vi "ReadPoints.vi"(8 "error in (no error)":errorcluster caption="错误输入（无错误）", 10 "工站":string, 11 "机种":string) -> (0 "error out":errorcluster caption="错误输出", 1 "Calcu":dbl[](array[numeric]), 2 "points":dbl[][](array[numeric]), 3 "Robot":cluster{"X":dbl, "Y":dbl}, 4 "RefMove":cluster{"X":dbl, "Y":dbl}, 5 "参考位":string)   [LabVIEW 2016]
uses:
  <vilib>/Utility/config.llb/Read Key (String).vi
  <vilib>/Utility/config.llb/NI_LVConfig.lvlib
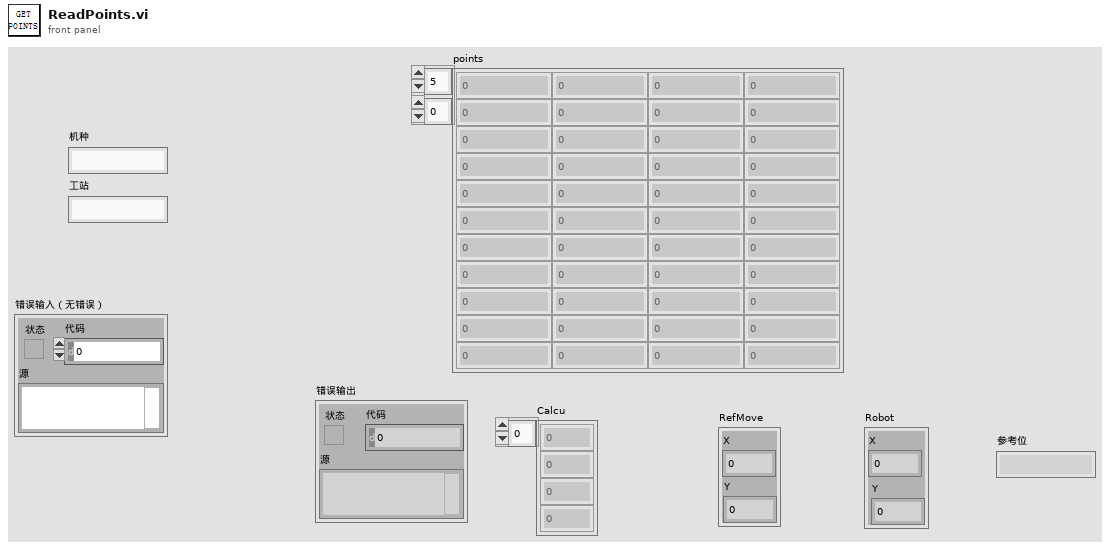
[diagram p1: front panel]
types:
  T1 = typedef "NI_LVConfig.lvlib/Config Data RefNum.ctl" = refnum<k1>
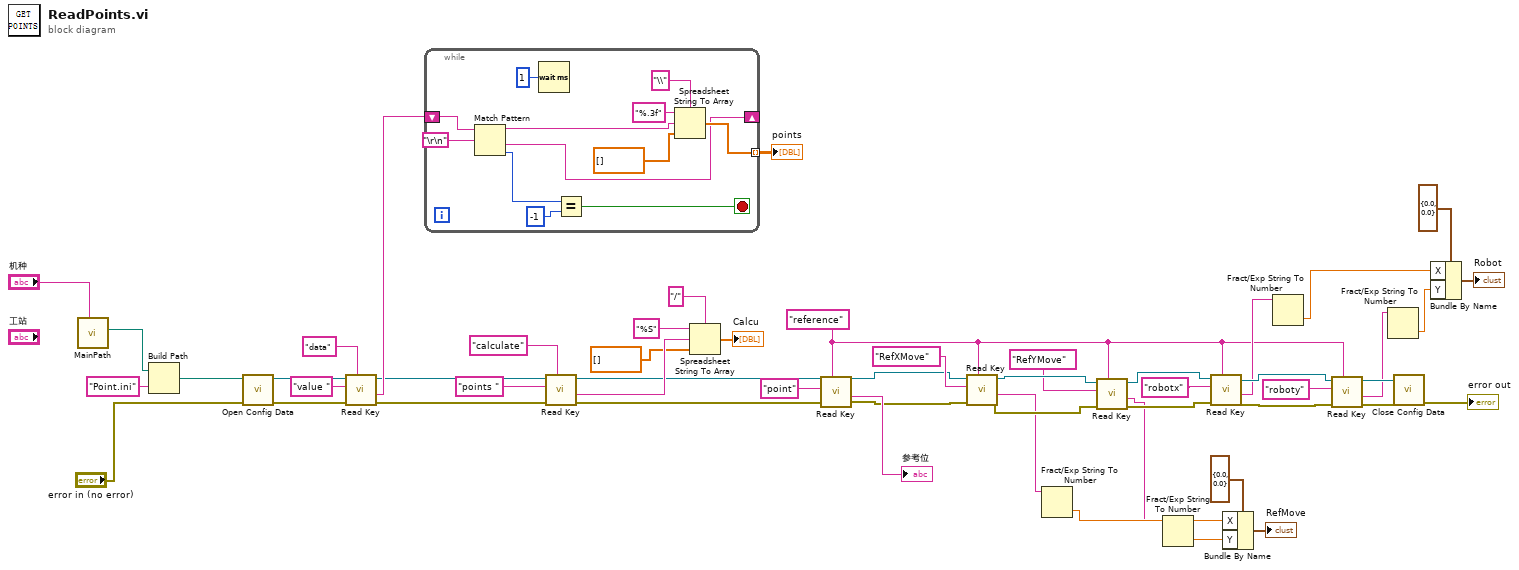
[diagram p0: block diagram]
diagram:
  w7 = "reference" ("section")
  n1 = call "MainPath.vi"("机种"="机种") -> ("路径"=w52:path)  [unwired: 9 in, 1 out]
  n2 = Build Path(base path=w52, name or relative path="Point.ini" ("名称或相对路径")) -> (appended path=w50:path)
  n3 = call <vilib>:"Open Config Data.vi"("error in (no error)"="error in (no error)", "configuration file path"=w50) -> ("error out"=w46:errorcluster, "refnum"=w47:T1)  [unwired: 7 in, 1 out]
  n4 = call-poly <vilib>:"Read Key.vi"("section"="data", "error in (no error)"=w46, "key"="value ", "refnum"=w47) -> ("error out"=w40:errorcluster, "value"=w43:string, "refnum out"=w41:T1)  [unwired: 4 in, 1 out]
  n5 = while {
    tunnel: [w56] -> w33 mode=indexing
    shift-right: [w54] -> _
    shift-left: w43 -> [w61]
    stop <- w55 stop-if-true
    n6 = Match Pattern(string=w61, regular expression="\r\n") -> (before substring=w59:string, after substring=w54:string, offset past match=w58:i32)  [unwired: 1 in, 1 out]
    n7 = Wait (ms)(milliseconds to wait=u32 1 ("等待时间（毫秒）")) -> ()  [unwired: 1 out]
    n8 = Equal?(x=w58, y=-1) -> (x = y?=w55:bool)
    n9 = Spreadsheet String To Array(delimiter (Tab)="\\" ("分隔符(Tab)"), format string="%.3f" ("格式字符串"), spreadsheet string=w59, array type (2D Dbl)=dbl[] []) -> (array=w56:dbl[])
  }
  "points" <- w33
  n10 = call-poly <vilib>:"Read Key.vi"("section"="calculate", "error in (no error)"=w40, "key"="points ", "refnum"=w41) -> ("error out"=w30:errorcluster, "value"=w37:string, "refnum out"=w31:T1)  [unwired: 4 in, 1 out]
  n11 = Spreadsheet String To Array(delimiter (Tab)="/" ("分隔符(Tab)"), format string="%S" ("格式字符串"), spreadsheet string=w37, array type (2D Dbl)=dbl[] []) -> (array=→"Calcu":dbl[])
  n12 = call-poly <vilib>:"Read Key.vi"("section"=w7, "error in (no error)"=w30, "key"="point", "refnum"=w31) -> ("error out"=w14:errorcluster, "value"=→"参考位":string, "refnum out"=w13:T1)  [unwired: 4 in, 1 out]
  n13 = call-poly <vilib>:"Read Key.vi"("section"=w7, "error in (no error)"=w14, "key"="RefXMove", "refnum"=w13) -> ("error out"=w12:errorcluster, "value"=w4:string, "refnum out"=w11:T1)  [unwired: 4 in, 1 out]
  n14 = Fract/Exp String To Number(string=w4) -> (number=w3:dbl)  [unwired: 3 in, 1 out]
  n15 = call-poly <vilib>:"Read Key.vi"("section"=w7, "error in (no error)"=w12, "key"="RefYMove", "refnum"=w11) -> ("error out"=w9:errorcluster, "value"=w2:string, "refnum out"=w10:T1)  [unwired: 4 in, 1 out]
  n16 = Fract/Exp String To Number(string=w2) -> (number=w1:dbl)  [unwired: 3 in, 1 out]
  n17 = call-poly <vilib>:"Read Key.vi"("section"=w7, "error in (no error)"=w9, "key"="robotx", "refnum"=w10) -> ("error out"=w26:errorcluster, "value"=w21:string, "refnum out"=w23:T1)  [unwired: 4 in, 1 out]
  n18 = Bundle By Name(cluster=cluster{"X":dbl, "Y":dbl} {"X"=0.0, "Y"=0.0} ("RefRobot"), "X"=w3, "Y"=w1) -> (→"RefMove":cluster{"X":dbl, "Y":dbl})
  n19 = Fract/Exp String To Number(string=w21) -> (number=w18:dbl)  [unwired: 3 in, 1 out]
  n20 = call-poly <vilib>:"Read Key.vi"("section"=w7, "error in (no error)"=w26, "key"="roboty", "refnum"=w23) -> ("error out"=w25:errorcluster, "value"=w20:string, "refnum out"=w24:T1)  [unwired: 4 in, 1 out]
  n21 = Fract/Exp String To Number(string=w20) -> (number=w17:dbl)  [unwired: 3 in, 1 out]
  n22 = call <vilib>:"Close Config Data.vi"("error in (no error)"=w25, "refnum"=w24) -> ("error out"=→"error out":errorcluster)  [unwired: 8 in, 1 out]
  n23 = Bundle By Name(cluster=cluster{"X":dbl, "Y":dbl} {"X"=0.0, "Y"=0.0} ("RefRobot"), "X"=w18, "Y"=w17) -> (→"Robot":cluster{"X":dbl, "Y":dbl})
